vi "Configure Trigger share.vi"(8 "error in":errorcluster, 9 "RX trigger options":T1 {"delay" format="%.0p"}, 10 "TX trigger options":T1 {"delay" format="%.0p"}, 11 "session in":T4[](array[typedef]) {"rx baseband session"."3630 session"."Address Space" items=["VXI/VME A16"=1, "VXI/VME A24"=2, "VXI/VME A32"=3, "VXI/VME A64"=4, "PXI Memory Allocations"=9, "PXI Configuration"=10, "PXI BAR0"=11, "PXI BAR1"=12, "PXI BAR2"=13, "PXI BAR3"=14, "PXI BAR4"=15, "PXI BAR5"=16]; "tx baseband session"."3610 session"."Address Space" items=["VXI/VME A16"=1, "VXI/VME A24"=2, "VXI/VME A32"=3, "VXI/VME A64"=4, "PXI Memory Allocations"=9, "PXI Configuration"=10, "PXI BAR0"=11, "PXI BAR1"=12, "PXI BAR2"=13, "PXI BAR3"=14, "PXI BAR4"=15, "PXI BAR5"=16]}) -> (0 "error out":errorcluster, 1 "actual rx delay":dbl, 2 "actual tx delay":dbl, 3 "session out":T4[](array[typedef]) {"rx baseband session"."3630 session"."Address Space" items=["VXI/VME A16"=1, "VXI/VME A24"=2, "VXI/VME A32"=3, "VXI/VME A64"=4, "PXI Memory Allocations"=9, "PXI Configuration"=10, "PXI BAR0"=11, "PXI BAR1"=12, "PXI BAR2"=13, "PXI BAR3"=14, "PXI BAR4"=15, "PXI BAR5"=16]; "tx baseband session"."3610 session"."Address Space" items=["VXI/VME A16"=1, "VXI/VME A24"=2, "VXI/VME A32"=3, "VXI/VME A64"=4, "PXI Memory Allocations"=9, "PXI Configuration"=10, "PXI BAR0"=11, "PXI BAR1"=12, "PXI BAR2"=13, "PXI BAR3"=14, "PXI BAR4"=15, "PXI BAR5"=16]})   [LabVIEW 2019]
uses:
  TypeDefs/Session.ctl
  <instrlib>/niMmWave/ni3620/Config/v1/Host/Public/High-Level/niMmWave Session.ctl
  <instrlib>/_niInstr/Register Bus/v0/Host/Public/Register Bus Session.ctl
  <instrlib>/_niInstr/Register Bus/v0/Host/Private/Session Data.ctl
  <instrlib>/niMmWave/ni3620/Config/v1/Host/Public/Typedefs/Board Information.ctl
  <instrlib>/niMmWave/ni3620/Config/v1/Host/Public/Typedefs/Hardware Revision.ctl
  <instrlib>/niMmWave/ni3620/Config/v1/Host/Public/Typedefs/Gain Mapping.ctl
  <instrlib>/niMmWave/ni3620/Config/v1/Host/Public/Typedefs/Correction Data.ctl
  <instrlib>/niMmWave/ni3620/Config/v1/Host/Public/Typedefs/Opera Characterization.ctl
  <instrlib>/niMmWave/ni3620/Config/v1/Host/Public/Corrections/Typedefs/Opera Characterization Main Header.ctl
  <instrlib>/niMmWave/ni3620/Config/v1/Host/Public/Corrections/Typedefs/Opera IF Board Information.ctl
  <instrlib>/niMmWave/ni3620/Config/v1/Host/Public/Corrections/Typedefs/Opera Characterization Instance Header.ctl
  <instrlib>/niMmWave/ni3620/Config/v1/Host/Public/Corrections/Typedefs/Opera Characterization Device Data Header.ctl
  <instrlib>/niMmWave/ni3620/Config/v1/Host/Public/Corrections/Typedefs/Opera LO Characterization Data Header.ctl
  <instrlib>/niMmWave/ni3620/Config/v1/Host/Public/Corrections/Typedefs/Opera IF Board Characterization Data Header.ctl
  <instrlib>/niMmWave/ni3620/Config/v1/Host/Public/Corrections/Typedefs/Opera Characterization Device Data.ctl
  <instrlib>/niMmWave/ni3620/Config/v1/Host/Public/Corrections/Typedefs/Opera LO2 Board Characterization Data.ctl
  <instrlib>/niMmWave/ni3620/Config/v1/Host/Public/Corrections/Typedefs/Opera LO Characterization Data.ctl
  <instrlib>/niMmWave/ni3620/Config/v1/Host/Public/Corrections/Typedefs/Opera IF Board Characterization Data.ctl
  <instrlib>/niMmWave/ni3620/Config/v1/Host/Public/Corrections/Typedefs/Opera IQ Impairment Data.ctl
  <instrlib>/niMmWave/ni3620/Config/v1/Host/Public/Typedefs/mmWave Adapter Session Data.ctl
  <instrlib>/niMmWave/ni3620/Config/v1/Host/Public/Typedefs/mmWave Adapter Data.ctl
  <instrlib>/niMmWave/ni3620/Config/v1/Host/Public/Typedefs/mmWave Adapter 2.ctl
  <instrlib>/niMmWave/ni3620/Config/v1/Shared/Typedefs/Subsystem ID.ctl
  <instrlib>/niMmWave/ni3620/Config/v1/Host/Public/Typedefs/mmWave Adapter Channel Information.ctl
  <instrlib>/niMmWave/ni3620/Config/v1/Host/Public/Typedefs/Temperature Coefficients.ctl
  <instrlib>/niMmWave/ni3620/Config/v1/Host/Public/Typedefs/mmWave Characterization.ctl
  <instrlib>/niMmWave/ni3620/Config/v1/Host/Public/Corrections/Typedefs/mmWave Characterization Main Header.ctl
  <instrlib>/niMmWave/ni3620/Config/v1/Host/Public/Corrections/Typedefs/mmWave Characterization Instance Header.ctl
  <instrlib>/niMmWave/ni3620/Config/v1/Host/Public/Typedefs/Session Cache.ctl
  <instrlib>/niMmWave/ni3620/Config/v1/Host/Public/Typedefs/LO2 settings cache.ctl
  <instrlib>/niMmWave/ni3620/Config/v1/Host/Public/Typedefs/LO2 source.ctl
  <instrlib>/niMmWave/ni3620/Config/v1/Host/Public/Typedefs/Desired and Coerced.ctl
  <instrlib>/niMmWave/ni3620/Config/v1/Host/Public/Typedefs/Export cache.ctl
  <instrlib>/niMmWave/ni3620/Config/v1/Host/Public/Typedefs/Path cache.ctl
  <instrlib>/niMmWave/ni3620/Config/v1/Host/Public/Typedefs/Daughterboard Type.ctl
  <instrlib>/niMmWave/ni3620/Config/v1/Host/Public/Typedefs/LO1 settings cache.ctl
  <instrlib>/niMmWave/ni3620/Config/v1/Host/Public/Typedefs/LO1 Source.ctl
  <instrlib>/niMmWave/ni3620/Config/v1/Host/Public/Typedefs/mmWave export cache.ctl
  <instrlib>/niMmWave/ni3620/Config/v1/Host/Private/Board/LO2/LO2 Board Configuration Cache.ctl
  <instrlib>/niMmWave/ni3620/Config/v1/Host/Public/Typedefs/reference clock routing settings.ctl
  <instrlib>/niMmWave/ni3620/Config/v1/Host/Public/Typedefs/LO2 routing settings.ctl
  <instrlib>/niMmWave/ni3620/Config/v1/Host/Private/Board/LO1/LO1 Board Configuration Cache.ctl
  <instrlib>/niMmWave/ni3620/Config/v1/Host/Public/Typedefs/LO1 source settings.ctl
  <instrlib>/niMmWave/ni3620/Config/v1/Host/Public/Typedefs/LO1 export settings.ctl
  <instrlib>/niMmWave/ni3620/Config/v1/Host/Public/Typedefs/LO1 mmWave settings.ctl
  TypeDefs/Tx Baseband Session.ctl
  <instrlib>/niMmWave/ni3610 and ni3630/controls/public/Main Settings.ctl
  <vilib>/Instr/_visa.llb/VISA Register Access Address Space.ctl
  <instrlib>/niMmWave/ni3610 and ni3630/controls/public/Register Adresses.ctl
  <instrlib>/niMmWave/ni3610 and ni3630/controls/public/Base Card Type.ctl
  <instrlib>/niMmWave/ni3610 and ni3630/controls/private/IQ Card Revision.ctl
  <instrlib>/niMmWave/ni3610 and ni3630/controls/public/Board Capability.ctl
  TypeDefs/Blank FPGA Reference.ctl
  TypeDefs/Rx Baseband Session.ctl
  TypeDefs/Hardware Configuration.ctl
  TypeDefs/Direction.ctl
  TypeDefs/Gain Ranging.ctl
  TypeDefs/PXI Trigger Bus Info.ctl
  TypeDefs/TX trigger config.ctl
  FPGA/SubVIs/Utility/FPGA driver trigger source.ctl
  FPGA/SubVIs/Utility/FPGA driver trigger destination.ctl
  TypeDefs/TX driver FPGA ref.ctl
  TypeDefs/RX driver FPGA ref.ctl
  <vilib>/Utility/error.llb/Error Cluster From Error Code.vi
  <vilib>/rvi/errors/niLvFpgaAdjustHostInterfaceError.vi
  <vilib>/rvi/interface/nirviReadWriteControl/nirviReadWriteControl.xnode
  NiFpgaLv.dll
  <vilib>/rvi/interface/Simulation/niFpgaSimulationCallBeginRW.vi
  <instrlib>/niMmWave/ni3620/Config/v1/Host/niMmWave Config v1 Host.lvlib
  <instrlib>/niMmWave/ni3620/Config/v1/Shared/niMmWave Config v1 Shared.lvlib
  <instrlib>/_niInstr/Register Bus/v0/Host/niInstr Register Bus v0 Host.lvlib
  <instrlib>/niMmWave/ni3610 and ni3630/ni3610_and_ni3630_Driver_Lib.lvlib
  FPGA/SubVIs/Utility/FPGA Utility.lvlib
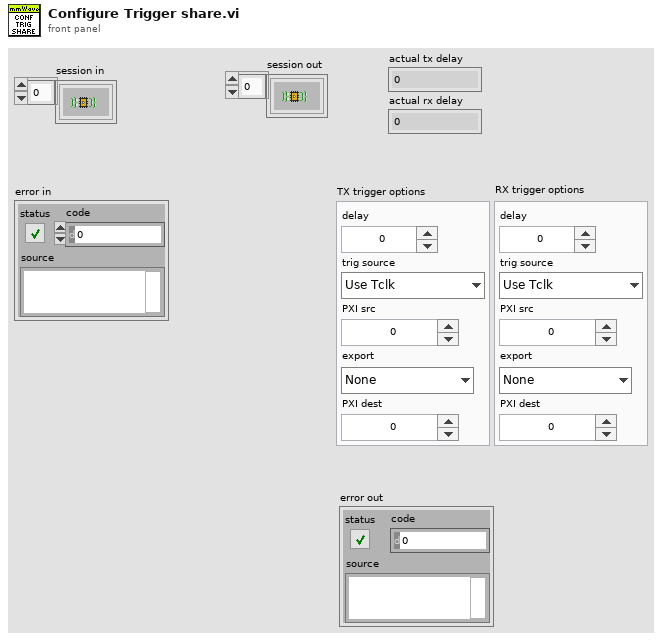
[diagram p1: front panel]
types:
  T1 = typedef "TX trigger config.ctl" = cluster{"delay":dbl, "trig source":T2, "PXI src":i32, "export":T3, "PXI dest":i32}
  T2 = typedef "FPGA Utility.lvlib/FPGA driver trigger source.ctl" = enum16{"Use Tclk", "PXI_Trig", "Aurora RX trig"}
  T3 = typedef "FPGA Utility.lvlib/FPGA driver trigger destination.ctl" = enum16{"None", "Source trig", "Synced trig", "Delayed sync"}
  T4 = typedef "Session.ctl" = cluster{"3620 session":refnum<queue>, "tx baseband session":T5, "rx baseband session":T13, "tx gain (dB)":dbl, "rx gain (dB)":dbl, "hardware configuration":T14, "gain ranging":T16[], "pxi trigger bus information":T17}
  T5 = typedef "Tx Baseband Session.ctl" = cluster{"3610 session":T6, "7902 reference":T12}
  T6 = typedef "ni3610_and_ni3630_Driver_Lib.lvlib/Main Settings.ctl" = cluster{"VISA resource name":refnum<visa-resource-name>, "Address Space":T7, "window_offset":u32, "register_addresses":T8, "required_MM_fpga_version":cluster{"signature":u32, "hardware":u32, "current revision":u32, "oldest revision":u32}, "CPLD Oldest Compat Version ":cluster{"hardware":u32, "CPLD firmware":u32}, "MM_FPGA_image_location":string, "is_init":bool, "card_type":T9, "DacLmkConfigFileName":string, "AdcLmkConfigFileName":string, "AdcConfigFileName":string, "DacConfigFileName_RevA":string, "DacConfigFileName_RevB":string, "Mulde hardware revision":u8, "bypass DAC PLL\n":bool, "IQ Card Revision":T10, "board capability":T11}
  T7 = typedef "VISA Register Access Address Space.ctl" = u16
  T8 = typedef "ni3610_and_ni3630_Driver_Lib.lvlib/Register Adresses.ctl" = cluster{"MM based Registers":cluster{"Revision":u32, "OldestCompatRev":u32, "signature":u32, "scratch":u32, "LedControl":u32, "BoardHwRev":u32, "BoardControl":u32, "ThermalStatus":u32, "BasebandStatus":u32, "BasebandControl":u32, "BasebandAuxSetup":u32, "BasebandAuxStatus":u32, "LmkSyncOutSetup":u32, " AdcSyncOutSetup":u32, " InjSyncOutSetup":u32, " PxiTrig0OutSetup":u32, " PxiTrig1OutSetup":u32, " PxiTrig2OutSetup":u32, " PxiTrig3OutSetup":u32, " PxiTrig4OutSetup":u32, " PxiTrig5OutSetup":u32, " PxiTrig6OutSetup":u32, " PxiTrig7OutSetup":u32}, "CPLD based Registers":cluster{"SlaveSignature":u32, "SlaveRevision":u32, "SlaveOldestCompatRev":u32, "SlaveScratch":u32, "SlaveSetup":u32, "SlaveStatus":u32, "IDacReg_offset":u32, "LMKRegGrp0_offset":u32, "QDacReg_offset":u32, "BrdTempSensorVal":u32, "TempSensorPowerDown":u32, "GPIOReg_offset":u32, "IAdcReg_offset":u32, "QAdcReg_offset":u32, "LMKRegGrp1_offset":u32, "QadcTempSensorVal":u32, "IadcTempSensorVal":u32, "RevisionReg":u32, "VcxoReg":u32, "CpldStatusReg":u32, "PowerReg":u32, "VBiasEnReg":u32, "ExtRefOeReg":u32, "QdacCtrlReg":u32, "QdacStatusReg":u32, "IdacCtrlReg":u32, "IdacStatusReg":u32, "QdacJtagIn":u32, "QdacJtagOut":u32, "IdacJtagIn":u32, "IdacJtagOut":u32, "IqDcSetupReg":u32, "QadcStatusReg":u32, "IadcStatusReg":u32, "BrdSetupReg":u32, "IqDcRevisionReg":u32, "PllStatusReg":u32, "EndpointScratchReg":u32, "AdcSyncCfgReg":u32, "IqCardOpampReg":u32}, "CPLD Register Offset":u32, "MM  Register Offset":u32, " PxiTrig0OutSetup":u32}
  T9 = typedef "ni3610_and_ni3630_Driver_Lib.lvlib/Base Card Type.ctl" = enum16{"unspecified", "ADC", "DAC"}
  T10 = typedef "ni3610_and_ni3630_Driver_Lib.lvlib/IQ Card Revision.ctl" = enum16{"RevA", "RevB", "RevC", "RevD"}
  T11 = typedef "ni3610_and_ni3630_Driver_Lib.lvlib/Board Capability.ctl" = cluster{"baseband sync":enum16{"no baseband sync", "baseband sync"}}
  T12 = typedef "Blank FPGA Reference.ctl" = refnum<k20>
  T13 = typedef "Rx Baseband Session.ctl" = cluster{"3630 session":T6, "7902 reference":T12}
  T14 = typedef "Hardware Configuration.ctl" = cluster{"direction":T15, "baseband only":bool}
  T15 = typedef "Direction.ctl" = enum16{"Transceiver", "Receiver", "Transmitter"}
  T16 = typedef "Gain Ranging.ctl" = cluster{"gain ranging active scope":string, "gain ranging stream session":refnum<k20>}
  T17 = typedef "PXI Trigger Bus Info.ctl" = cluster{"chassis resource name":refnum<visa-resource-name>, "7902R (TX)":i16, "3610 (TX)":i16, "3620 (IF)":i16, "3630 (RX)":i16, "7902R (RX)":i16}
  T18 = typedef "Constants.ctl" = cluster{"data clock rate (Hz)":dbl, "sample rate (Hz)":dbl, "sample rate selector string":string, "default tx bitfile path":path, "default rx bitfile path":path, "default proc bitfile path":path}
  T19 = typedef "RX driver FPGA ref.ctl" = refnum<k20>
  T20 = typedef "TX driver FPGA ref.ctl" = refnum<k20>
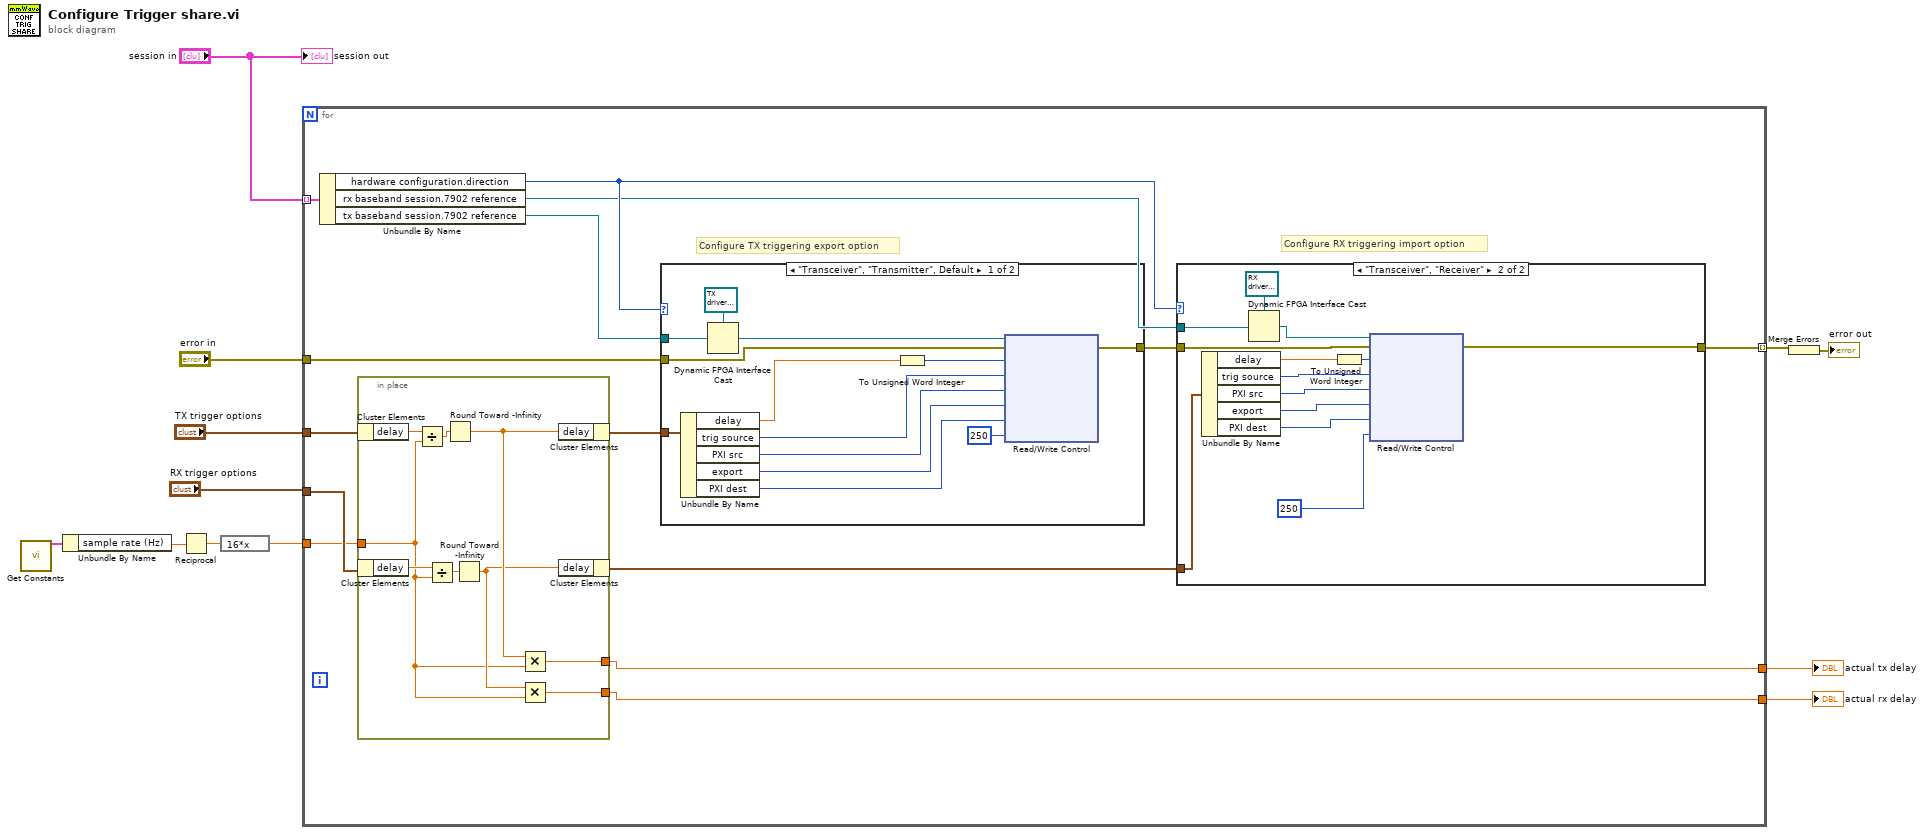
[diagram p0: block diagram]
diagram:
  n1 = call "Get Constants.vi"() -> ("constants"=w6:T18)  [unwired: 15 in]
  n2 = Unbundle By Name(w6) -> ("sample rate (Hz)"=w5:dbl)
  n3 = Reciprocal(x=w5) -> (1/x=w4:dbl)
  n4 = expression code="16*x"(w4) -> (w3:dbl)
  n5 = for {
    tunnel: "session in" -> [w26] mode=indexing
    tunnel: "error in" -> [w23]
    tunnel: [w20] -> w10 mode=indexing
    tunnel: "TX trigger options" -> [w19]
    tunnel: "RX trigger options" -> [w18]
    tunnel: w3 -> [w17]
    tunnel: [w14] -> w2
    tunnel: [w13] -> w1
    # "Configure RX triggering import option"
    # "Configure TX triggering export option"
    n6 = Unbundle By Name(w26) -> ("hardware configuration.direction"=w24:T15, "rx baseband session.7902 reference"=w22:T12, "tx baseband session.7902 reference"=w25:T12)
    n7 = in-place {
      in-place-border: w17 -> [w29]
      in-place-border: [w28] -> w14
      in-place-border: [w27] -> w13
      n8 = in-place-cluster #1(w19) -> ("delay"=w35:dbl)
      n9 = in-place-cluster #2(w18) -> ("delay"=w33:dbl)
      n10 = Divide(x=w35, y=w29) -> (x/y=w34:dbl)
      n11 = Divide(x=w33, y=w29) -> (x/y=w32:dbl)
      n12 = Round Toward -Infinity(1:w34) -> (0:w31:dbl)
      n13 = Round Toward -Infinity(1:w32) -> (0:w30:dbl)
      n14 = Multiply(x=w31, y=w29) -> (x*y=w27:dbl)
      n15 = Multiply(x=w30, y=w29) -> (x*y=w28:dbl)
      n16 = in-place-cluster #1("delay"=w31) -> (w16:T1)
      n17 = in-place-cluster #2("delay"=w30) -> (w15:T1)
    }
    n18 = case shown="\"Transceiver\", \"Transmitter\", Default" w24 {
      tunnel: w25 -> [w62 _]
      tunnel: w23 -> [w59 w63]
      tunnel: [w52 w63] -> w21
      tunnel: w16 -> [w58 _]
      frame "Transceiver", "Transmitter", Default {
        n19 = Unbundle By Name(w58) -> ("delay"=w51:dbl, "trig source"=w57:T2, "PXI src"=w56:i32, "export"=w55:T3, "PXI dest"=w54:i32)
        n20 = Dynamic FPGA Interface Cast(Session In=T20 refnum ("Type"), Type=w62) -> (Session Out=w60:T20)
        n21 = To Unsigned Word Integer(number=w51) -> (unsigned 16bit integer=w50:u16)
        n22 = xnode "Read/Write Control"("FPGA VI Reference In"=w60, "error in"=w59, "trig.delay"=w50, "trig.source"=w57, "trig.pxi src"=w56, "trig.export"=w55, "trig.pxi dst"=w54, "trig.export dur"=u32 250 ("trig.dur")) -> ("error out"=w52:errorcluster)  [unwired: 1 out]
      }
      frame "Receiver" {
      }
    }
    n23 = case shown="\"Transceiver\", \"Receiver\"" w24 {
      tunnel: w22 -> [_ w49]
      tunnel: w21 -> [w36 w42]
      tunnel: [w36 w38] -> w20
      tunnel: w15 -> [_ w41]
      frame "Transmitter", Default {
      }
      frame "Transceiver", "Receiver" {
        n24 = Unbundle By Name(w41) -> ("delay"=w44:dbl, "trig source"=w45:T2, "PXI src"=w46:i32, "export"=w39:T3, "PXI dest"=w47:i32)
        n25 = Dynamic FPGA Interface Cast(Session In=T19 refnum ("Type"), Type=w49) -> (Session Out=w43:T19)
        n26 = To Unsigned Word Integer(number=w44) -> (unsigned 16bit integer=w37:u16)
        n27 = xnode "Read/Write Control"("FPGA VI Reference In"=w43, "error in"=w42, "trig.delay"=w37, "trig.source"=w45, "trig.pxi src"=w46, "trig.export"=w39, "trig.pxi dst"=w47, "trig.export dur"=u32 250 ("trig.dur")) -> ("error out"=w38:errorcluster)  [unwired: 1 out]
      }
    }
  }
  "actual tx delay" <- w1
  "actual rx delay" <- w2
  n28 = Merge Errors(w10) -> (→"error out":errorcluster)
  "session out" <- "session in"
